vi "CANOpen_Search Channel Ref.vi"(8 "error in (no error)":errorcluster, 9 "GUID":string, 10 "Section Ref in":T1 format="%.0x", 11 "Device Ref":T1 format="%.0x") -> (0 "error out":errorcluster, 2 "Found":bool, 3 "Channel Data Reference":T2 format="%.0x")   [LabVIEW 2021, in "CANOpen Addon Engine.lvlib"]
uses:
  <vilib>/NI VeriStand/Custom Device API/Custom Device Item Ref.ctl
  <vilib>/NI VeriStand/Custom Device API/Data Reference.ctl
  <vilib>/NI VeriStand/Custom Device API/Data Access Type.ctl
  <vilib>/NI VeriStand/Custom Device Tools/Custom Device Utility Library/NI VeriStand - Search for Item by GUID.vi
  CANOpen Addon Engine.lvlib
  <vilib>/NI VeriStand/Custom Device Tools/Custom Device Utility Library/Custom Device Utility Library.lvlib
  <vilib>/NI VeriStand/Custom Device API/Custom Device API.lvlib
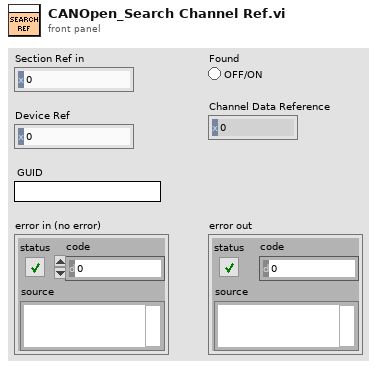
[diagram p1: front panel]
types:
  T1 = typedef "Custom Device API.lvlib/Custom Device Item Ref.ctl" = u64
  T2 = typedef "Custom Device API.lvlib/Data Reference.ctl" = i32
  T3 = typedef "Custom Device API.lvlib/Data Access Type.ctl" = enum16{"Read", "Write"}
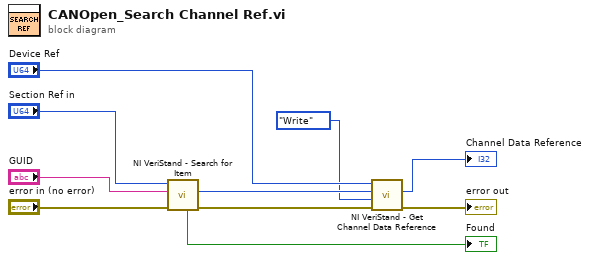
[diagram p0: block diagram]
diagram:
  n1 = call-poly <vilib>:"NI VeriStand - Search for Item.vi"("error in"="error in (no error)", "Item GUID"="GUID", "Section Ref in"="Section Ref in") -> ("error out"=w6:errorcluster, "Item Ref"=w8:T1, "Found"=→"Found":bool)  [unwired: 5 in, 1 out]
  n2 = call <vilib>:"NI VeriStand - Get Channel Data Reference.vi"("error in (no error)"=w6, "Access"=Data_Access_Type."Write", "Channel Ref in"=w8, "Device Ref in"="Device Ref") -> ("error out"=→"error out":errorcluster, "Channel Data Reference"=→"Channel Data Reference":T2)  [unwired: 5 in, 1 out]
